vi "-8340 No File--error.vi"(8 "error in (no error)":errorcluster, 11 "File Path":string) -> (0 "error out":errorcluster, 2 "Error Code":i32)   [LabVIEW 2019, in "Open Xml.lvlib"]
uses:
  Open Xml.lvlib
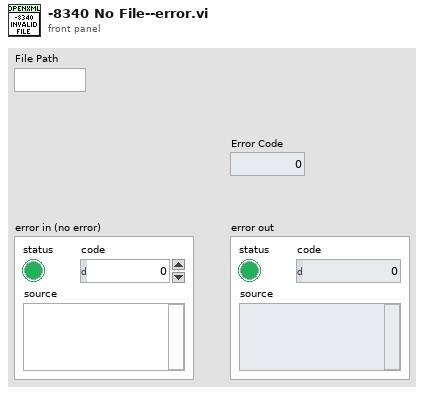
[diagram p1: front panel]
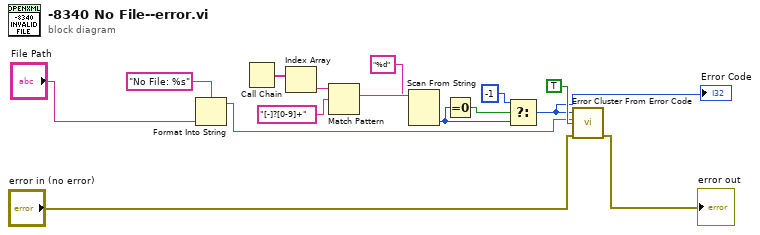
[diagram p0: block diagram]
diagram:
  n1 = Format Into String(format string="No File: %s" ("source"), "File Path") -> (resulting string=w10:string)  [unwired: 2 in, 1 out]
  n2 = Call Chain() -> (call chain=w12:string[])
  n3 = Index Array(array=w12) -> (element=w4:string)  [unwired: 1 in]
  n4 = Match Pattern(string=w4, regular expression="[-]?[0-9]+") -> (match substring=w3:string)  [unwired: 1 in, 3 out]
  n5 = Scan From String(format string="%d", input string=w3) -> (output 1=w7:i32)  [unwired: 3 in, 3 out]
  n6 = Equal To 0?(x=w7) -> (x = 0?=w6:bool)
  n7 = Select(t=-1, s=w6, f=w7) -> (s? t:f=w1:i32)
  "Error Code" <- w1
  n8 = call <vilib>:"Error Cluster From Error Code.vi"("show call chain? (False)"=TRUE, "error in (no error)"="error in (no error)", "error message (\"\")"=w10, "error code (0)"=w1) -> ("error out"=→"error out":errorcluster)  [unwired: 5 in]
